vi "Test1.vi"   [LabVIEW 2013]
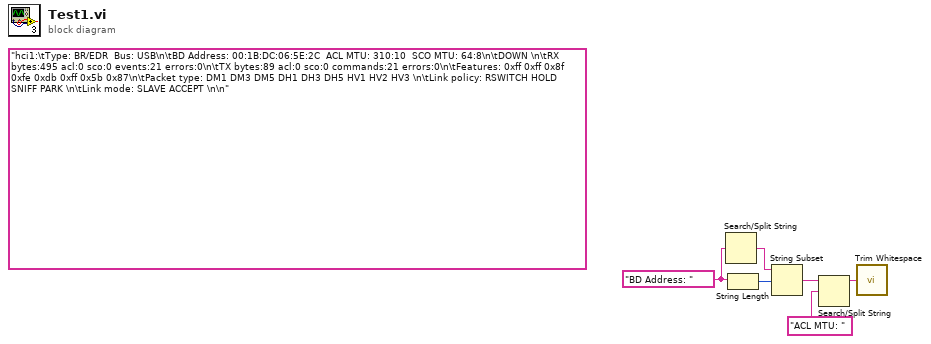
[diagram p0: block diagram]
diagram:
  w4 = "BD Address: " ("search string/char (-)")
  (unwired) "hci1:\tType: BR/EDR  Bus: USB\n\tBD Address: 00:1B:DC:06:5E:2C  ACL MTU: 310:10  SCO MTU: 64:8\n\tDOWN \n\tRX bytes:495 acl:0 sco:0 events:21 errors:0\n\tTX bytes:89 acl:0 sco:0 commands:21 errors:0\n\tFeatures: 0xff 0xff 0x8f 0xfe 0xdb 0xff 0x5b 0x87\n\tPacket type: DM1 DM3 DM5 DH1 DH3 DH5 HV1 HV2 HV3 \n\tLink policy: RSWITCH HOLD SNIFF PARK \n\tLink mode: SLAVE ACCEPT \n\n"
  n1 = Search/Split String(search string/char (-)=w4) -> (match + rest of string=w5:string)  [unwired: 2 in, 2 out]
  n2 = String Length(string=w4) -> (length=w2:i32)
  n3 = String Subset(string=w5, offset (0)=w2) -> (substring=w3:string)  [unwired: 1 in]
  n4 = Search/Split String(string=w3, search string/char (-)="ACL MTU: ") -> (substring before match=w1:string)  [unwired: 1 in, 2 out]
  n5 = call <vilib>:"Trim Whitespace.vi"("string"=w1) -> ()  [unwired: 1 in, 1 out]
